vi "Global.vi"() -> ()   [LabVIEW 2011]
panel:
  in  "Stop":bool
  in  "Temp":dbl
  in  "Level":dbl
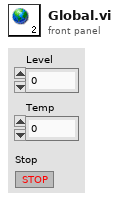
[diagram p1: front panel]
diagram:
